vi "Open Single Victor.vi"(7 "refnum name":string="TalonSRX", 8 "error in (no error)":errorcluster, 9 "Master Controller to Follow":T1={"DeviceStatus"={"status"=FALSE, "code"=0, "source"=""}, "Type"=enum."PWM", "PWM"={"PWM Channel"=enum."PWM 1", "DeadBand"={"Name"="", "maxPositivePwm"=0, "minPositivePwm"=0, "centerPwm"=0, "maxNegativePwm"=0, "minNegativePwm"=0, "angularRange"=0}}, "CAN"={"Device Number"=255, "SetOutput VI Ref"=variant(enum8{"Percent VBus", "Current", "Speed", "Position", "Voltage"} enum."Percent VBus"), "GetOutput VI Ref"=variant(refnum<k1> refnum), "Enable VI Ref"=variant(dbl 12.0), "Disable VI Ref"=variant(enum8{"Percent VBus", "Speed", "Position", "Slave", "Unchanged / Invalid", "Voltage Compensation", "Current", "Motion Profile"} enum."Percent VBus"), "Data"=variant}, "Invert"=FALSE, "DIO PWM"={"PWM \"Enable\" Channel"=enum."Invalid", "DIOChannel"=enum."Invalid", "PWM Rate"=0.0}}, 10 "Device Number":u8, 11 "Invert?":bool) -> (0 "error out":errorcluster)   [LabVIEW 2019, in "Drive.lvlib" / "TalonSRX.lvclass"]
doc: "This VI configures a Victor SPX with the standards normally used by the Howdy Bots."
uses:
  TalonSRX.lvclass
  <vilib>/Rock Robotics/WPI/MotorControl/WPI_MotorControlDeviceRef.ctl
  <vilib>/Rock Robotics/WPI/MotorControl/WPI_MotorControlType.ctl
  <vilib>/Rock Robotics/SystemInterfaces/DIO/FPGA_DIOPWMChannel.ctl
  <vilib>/Rock Robotics/WPI/PWM/WPI_PWMDeadband.ctl
  <vilib>/Rock Robotics/SystemInterfaces/DIO/FPGA_DIOChannel.ctl
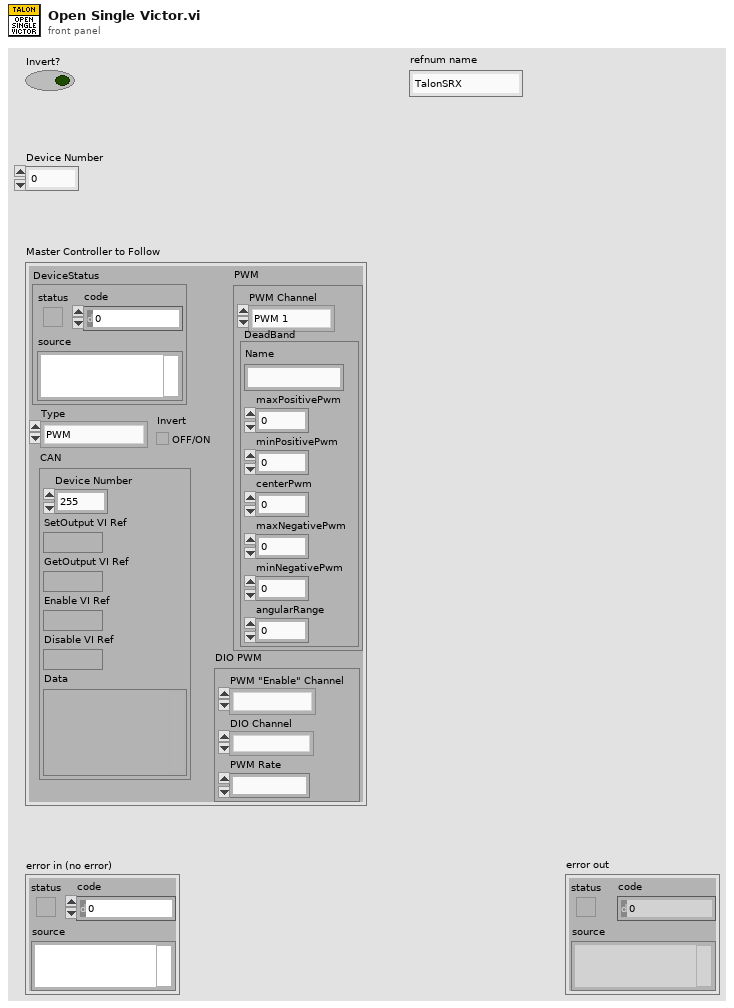
[diagram p1: front panel]
types:
  T1 = typedef "WPI_MotorControlDeviceRef.ctl" = cluster{"DeviceStatus":errorcluster, "Type":T2, "PWM":cluster{"PWM Channel":T3, "DeadBand":T4}, "CAN":cluster{"Device Number":u8, "SetOutput VI Ref":variant, "GetOutput VI Ref":variant, "Enable VI Ref":variant, "Disable VI Ref":variant, "Data":variant}, "Invert":bool, "DIO PWM":cluster{"PWM \"Enable\" Channel":T3, "DIOChannel":T5, "PWM Rate":dbl}}
  T2 = typedef "WPI_MotorControlType.ctl" = enum16{"PWM", "CAN", "DIO PWM"}
  T3 = typedef "FPGA_DIOPWMChannel.ctl" = enum8{"PWM 0", "PWM 1", "PWM 2", "PWM 3", "PWM 4", "PWM 5", "PWM 6", "PWM 7", "PWM 8", "PWM 9", "PWM MXP 0", "PWM MXP 1", "PWM MXP 2", "PWM MXP 3", "PWM MXP 4", "PWM MXP 5", "PWM MXP 6", "PWM MXP 7", "PWM MXP 8", "PWM MXP 9", "Invalid"}
  T4 = typedef "WPI_PWMDeadband.ctl" = cluster{"Name":string, "maxPositivePwm":i32, "minPositivePwm":i32, "centerPwm":i32, "maxNegativePwm":i32, "minNegativePwm":i32, "angularRange":u16}
  T5 = typedef "FPGA_DIOChannel.ctl" = enum8{"DIO 0", "DIO 1", "DIO 2", "DIO 3", "DIO 4", "DIO 5", "DIO 6", "DIO 7", "DIO 8", "DIO 9", "DIO MXP 0", "DIO MXP 1", "DIO MXP 2", "DIO MXP 3", "DIO MXP 4", "DIO MXP 5", "DIO MXP 6", "DIO MXP 7", "DIO MXP 8", "DIO MXP 9", "DIO MXP 10", "DIO MXP 11", "DIO MXP 12", "DIO MXP 13", "DIO MXP 14", "DIO MXP 15", "SPI Port CS1", "SPI Port CS2", "SPI Port CS3", "SPI Port MISO", "SPI Port MOSI", "Invalid"}
  T6 = enum16{"FollowerType_PercentOutput", "FollowerType_AuxOutput1"}
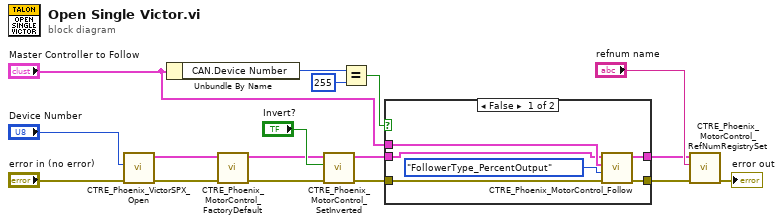
[diagram p0: block diagram]
diagram:
  n1 = call <vilib>:"CTRE_Phoenix_VictorSPX_Open.vi"("error in"="error in (no error)", "Device Number"="Device Number") -> ("error out"=w6:errorcluster, "CAN Talon SRX Ref"=w5:T1)  [unwired: 8 in]
  n2 = Unbundle By Name("Master Controller to Follow") -> ("CAN.Device Number"=w3:u8)
  n3 = call <vilib>:"CTRE_Phoenix_MotorControl_FactoryDefault.vi"("error in"=w6, "PhoenixMotorControlDevRef"=w5) -> ("error out"=w9:errorcluster, "PhoenixMotorControlDevRef"=w10:T1)  [unwired: 8 in]
  n4 = call <vilib>:"CTRE_Phoenix_MotorControl_SetInverted.vi"("error in (no error)"=w9, "Invert?"="Invert?", "PhoenixMotorControlDevRef"=w10) -> ("error out"=w13:errorcluster, "PhoenixMotorControlDevRef"=w12:T1)  [unwired: 7 in]
  n5 = Equal?(x=w3, y=u8 255) -> (x = y?=w1:bool)
  n6 = case shown="False" w1 {
    tunnel: [w23 w24] -> w16
    tunnel: [w22 w25] -> w14
    tunnel: w13 -> [w21 w24]
    tunnel: "Master Controller to Follow" -> [w20 _]
    tunnel: w12 -> [w19 w25]
    frame False {
      n7 = call <vilib>:"CTRE_Phoenix_MotorControl_Follow.vi"("error in (no error)"=w21, "FollowerType"=T6."FollowerType_PercentOutput", "Master Controller to Follow"=w20, "PhoenixMotorControlDevRef"=w19) -> ("error out"=w23:errorcluster, "PhoenixMotorControlDevRef"=w22:T1)  [unwired: 6 in]
    }
    frame True {
    }
  }
  n8 = call <vilib>:"CTRE_Phoenix_MotorControl_RefNumRegistrySet.vi"("error in (no error)"=w16, "refnum name"="refnum name", "PhoenixMotorControlDevRef"=w14) -> ("error out"=→"error out":errorcluster)  [unwired: 7 in, 1 out]
